vi "Test Serial Communication.vi"() -> ()   [LabVIEW 2015]
uses:
  Session/Raw FPGA/FPGA Session.lvclass
  Session/FPGA Serial Session.lvclass
  Reusable/Session APIs/File Access/Config Data/Config Data.lvclass
  Reusable/Session APIs/File Access/Config Data/Config Data.lvclass/Config Data.ctl
  Session/FPGA Serial Session.lvclass/FPGA Serial Session.ctl
  Reusable/Session APIs/File Access/Config Data/Accessors/Write Cfg Path.vi
  Session/Write fpgaSession.vi
  <userlib>/_Session Fwk/Session - Root.lvclass
panel:
  out "length":cluster{i32, i16}(graph)
  out "Missed Data":i32
  in  "repeat":bool
  in  "milliseconds to wait":u32=1000
  out "CMD Time":timestamp format="%<%H:%M:%S%2u>T"
  out "Close Error":errorcluster
  out "Config Error":errorcluster
  in  "Data":enum16{"PPT", "Vaisala", "TEC"}(ring)
  out "Data Error":errorcluster
  in  "DataIn":string
  in  "Stop":bool
  out "DataOut":string
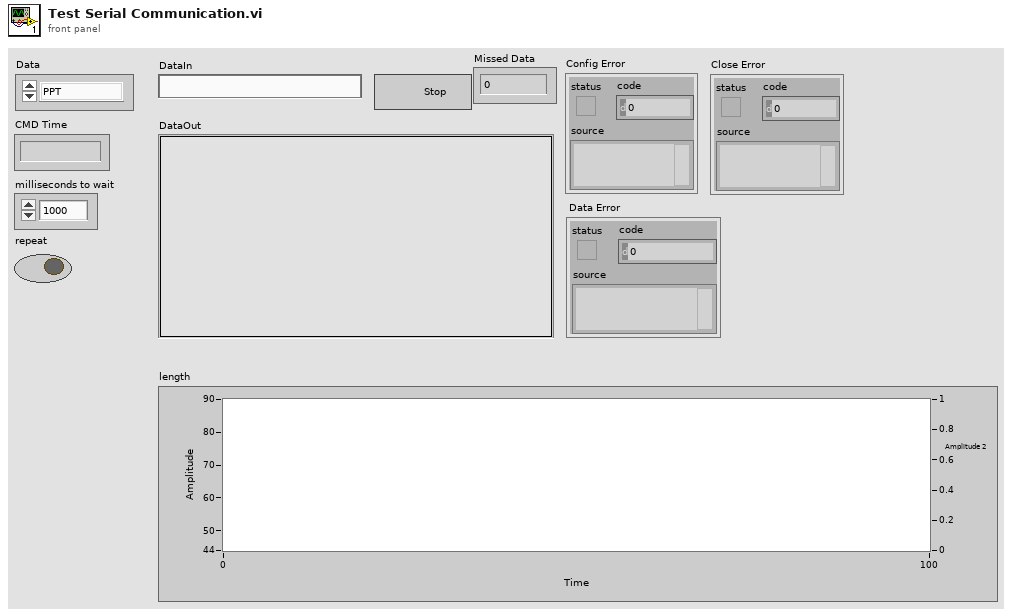
[diagram p1: front panel]
types:
  T1 = typedef "Session - Root.lvclass/Session Handle.ctl" = refnum<data-value>
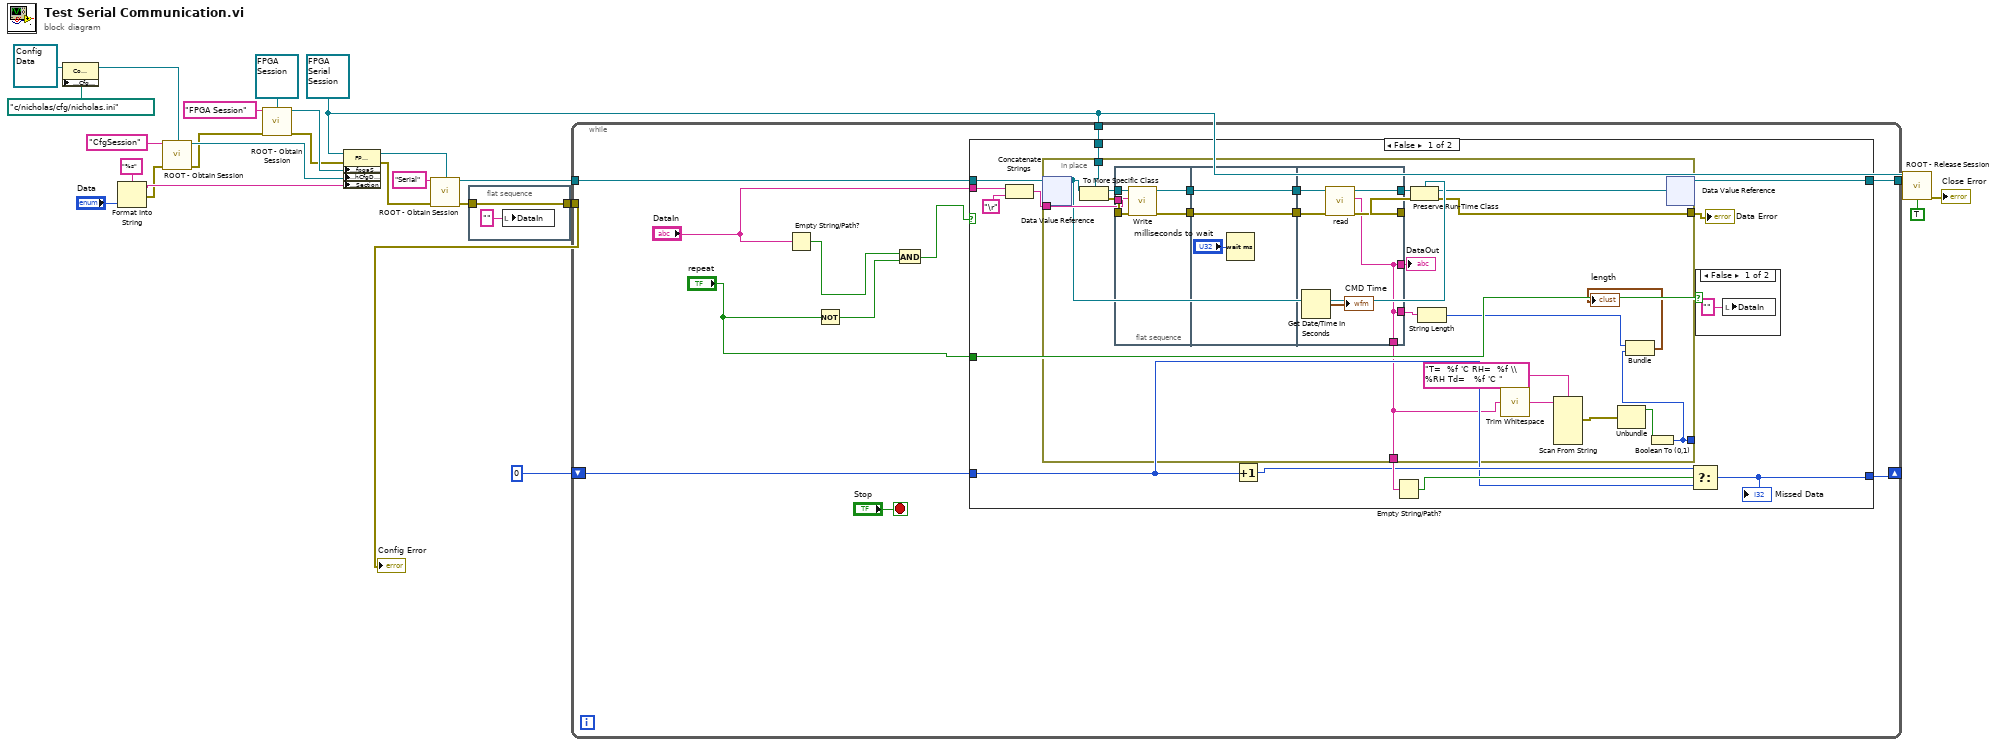
[diagram p0: block diagram]
diagram:
  w2 = refnum<class "FPGA Serial Session.lvclass"> refnum ("FPGA Serial Session.lvclass")
  n1 = property class="Config Data"(reference=refnum<class "Config Data.lvclass"> refnum ("Config Data"), "Accessors:Cfg Path"=path "c:/nicholas/cfg/nicholas.ini" ("Cfg Path")) -> (reference out=w18:refnum<class "Config Data.lvclass">)  [unwired: 1 in, 1 out]
  n2 = Format Into String(format string="%s", "Data") -> (resulting string=w12:string, error out=w6:errorcluster)  [unwired: 2 in]
  n3 = call <userlib>:"ROOT - Obtain Session.vi"("Session Name ()"="CfgSession", "OBJ - Session"=w18, "error in (no error)"=w6) -> ("Session Handle"=w16:T1, "error out"=w8:errorcluster)  [unwired: 10 in, 1 out]
  n4 = call <userlib>:"ROOT - Obtain Session.vi"("Session Name ()"="FPGA Session", "OBJ - Session"=refnum<class "FPGA Session.lvclass"> refnum ("FPGA Session"), "error in (no error)"=w8) -> ("Session Handle"=w23:T1, "error out"=w7:errorcluster)  [unwired: 10 in, 1 out]
  n5 = property class="FPGA Serial Session"(reference=w2, error in=w7, "Accessors:fpgaSession"=w23, "Accessors:hCfgData"=w16, "Accessors:Section"=w12) -> (reference out=w22:refnum<class "FPGA Serial Session.lvclass">, error out=w9:errorcluster)
  n6 = call <userlib>:"ROOT - Obtain Session.vi"("Session Name ()"="Serial", "OBJ - Session"=w22, "error in (no error)"=w9) -> ("Session Handle"=w15:T1, "error out"=w4:errorcluster)  [unwired: 10 in, 1 out]
  n7 = flat-sequence {
    tunnel: w4 -> [w26]
    tunnel: [w26] -> w3
    frame #0 {
      n8 = local write "DataIn"("" ("DataIn")) -> ()
    }
  }
  n9 = while {
    tunnel: w15 -> [w38]
    tunnel: [w36] -> w11
    tunnel: w3 -> [_]
    tunnel: w2 -> [w34]
    shift-right: [w28] -> _
    shift-left: 0 -> [w29]
    stop <- "Stop" stop-if-true
    n10 = Empty String/Path?(string/path="DataIn") -> (empty?=w32:bool)
    n11 = Not(x="repeat") -> (.not. x?=w31:bool)
    n12 = And(x=w32, y=w31) -> (x .and. y?=w30:bool)
    n13 = case shown="False" w30 {
      tunnel: w38 -> [w49 w91]
      tunnel: "DataIn" -> [w51 _]
      tunnel: [w45 w91] -> w36
      tunnel: w34 -> [w48 _]
      tunnel: "repeat" -> [w44 _]
      tunnel: w29 -> [w40 w90]
      tunnel: [w39 w90] -> w28
      frame False {
        n14 = Concatenate Strings(w51, "\r") -> (w47:string)
        n15 = in-place {
          in-place-border: w48 -> [w75]
          in-place-border: w47 -> [w70]
          in-place-border: [w62] -> w46
          in-place-border: [w58] -> w43
          in-place-border: [w55] -> _
          n16 = in-place-dvr #1(w49) -> (w65:refnum<class "Session - Root.lvclass">)  [unwired: 1 out]
          n17 = To More Specific Class(target class=w75, reference=w65) -> (specific class reference=w74:refnum<class "FPGA Serial Session.lvclass">, error out=w73:errorcluster)  [unwired: 1 in]
          n18 = flat-sequence {
            tunnel: w74 -> [w80]
            tunnel: w73 -> [w79]
            tunnel: [w78] -> w71
            tunnel: w70 -> [w77]
            tunnel: [w76] -> w67
            tunnel: [w83] -> w72
            tunnel: w71 -> [w83]
            tunnel: [w81] -> w68
            tunnel: w67 -> [w81]
            tunnel: w72 -> [w89]
            tunnel: [w84] -> w69
            tunnel: [w88] -> w63
            tunnel: w68 -> [w87]
            tunnel: [w86] -> w66
            tunnel: [w84] -> w58
            tunnel: [w84] -> w61
            frame #0 {
              n19 = call-dynamic "Write.vi"("error in"=w79, "Data In"=w77, "Text Session in"=w80) -> ("error out"=w76:errorcluster, "Text Session out"=w78:refnum<class "FPGA Serial Session.lvclass">)  [unwired: 7 in]
            }
            frame #1 {
              n20 = Wait (ms)(milliseconds to wait="milliseconds to wait") -> ()  [unwired: 1 out]
            }
            frame #2 {
              n21 = Get Date/Time In Seconds() -> (seconds since 1Jan1904=→"CMD Time":timestamp)
              n22 = call-dynamic "read.vi"("error in"=w87, "Text Session in"=w89) -> ("error out"=w88:errorcluster, "Data Out"=w84:string, "Text Session out"=w86:refnum<class "FPGA Serial Session.lvclass">)  [unwired: 7 in]
            }
          }
          n23 = Preserve Run-Time Class(object in=w66, error in=w63, 2:w65) -> (object out=w64:refnum<class "Session - Root.lvclass">, error out=w62:errorcluster)
          n24 = String Length(string=w61) -> (length=w54:i32)
          n25 = call <vilib>:"Trim Whitespace.vi"("string"=w58) -> ("trimmed string"=w59:string)  [unwired: 1 in]
          n26 = Scan From String(format string="T=  %f 'C RH=  %f \\%RH Td=   %f 'C ", input string=w59) -> (error out=w57:errorcluster)  [unwired: 8 in, 2 out]
          n27 = Unbundle(w57) -> ("status"=w56:bool)  [unwired: 2 out]
          n28 = Boolean To (0,1)(Boolean=w56) -> (0, 1=w55:i16)
          n29 = Bundle(w54, w55) -> (→"length":cluster{i32, i16})  [unwired: 1 in]
          n30 = in-place-dvr #1(w64) -> (w45:T1)  [unwired: 1 out]
          "DataOut" <- w69
        }
        "Data Error" <- w46
        n31 = Increment(x=w40) -> (x+1=w41:i32)
        n32 = Empty String/Path?(string/path=w43) -> (empty?=w42:bool)
        n33 = Select(t=w41, s=w42, f=w40) -> (s? t:f=w39:i32)
        "Missed Data" <- w39
        n34 = case shown="False" w44 {
          frame False {
            n35 = local write "DataIn"("" ("DataIn")) -> ()
          }
          frame True {
          }
        }
      }
      frame True {
      }
    }
  }
  n36 = call <userlib>:"ROOT - Release Session.vi"("OBJ - Session in"=w2, "Session Handle in"=w11, "force destroy? (F)"=TRUE) -> ("error out"=→"Close Error":errorcluster)  [unwired: 11 in, 1 out]
  "Config Error" <- w3
